vi "Oscilloscope_Analyzer.vi"(7 "Note":enum16{"Модулятор", "Команда", "Кадер", "Кодер"}(ring), 8 "error in (no error)":errorcluster, 11 "RFID system in":refnum<class "RFID system.lvclass">) -> (0 "error out":errorcluster, 3 "RFID system out":refnum<class "RFID system.lvclass">)   [LabVIEW 2019]
uses:
  <vilib>/express/express analysis/Spectral/XNode/ExpressSpectralMeasurementsBlockNode.xnode
  <vilib>/express/express analysis/Spectral/Block/exnSpectralBlock spectral measurements RMS poly.vi
  <vilib>/express/express analysis/Spectral/Block/exnSpectralBlock spectral measurements RMS WFM.vi
  Store.lvclass
  RFID system.lvclass
panel:
  in  "Tab Control":enum32{"Complex", "Real"}(tab)
  out "Osciloscope":cluster{"t0":dbl, "dt":dbl, "Y":dbl[]}(graph)
  out "Spectrum Analyzer":cluster{"t0":dbl, "dt":dbl, "Y":dbl[]}(graph)
  out "Osciloscope":waveform(dbl)(graph)
  out "Spectrum Analyzer":cluster{"t0":dbl, "dt":dbl, "Y":dbl[]}(graph)
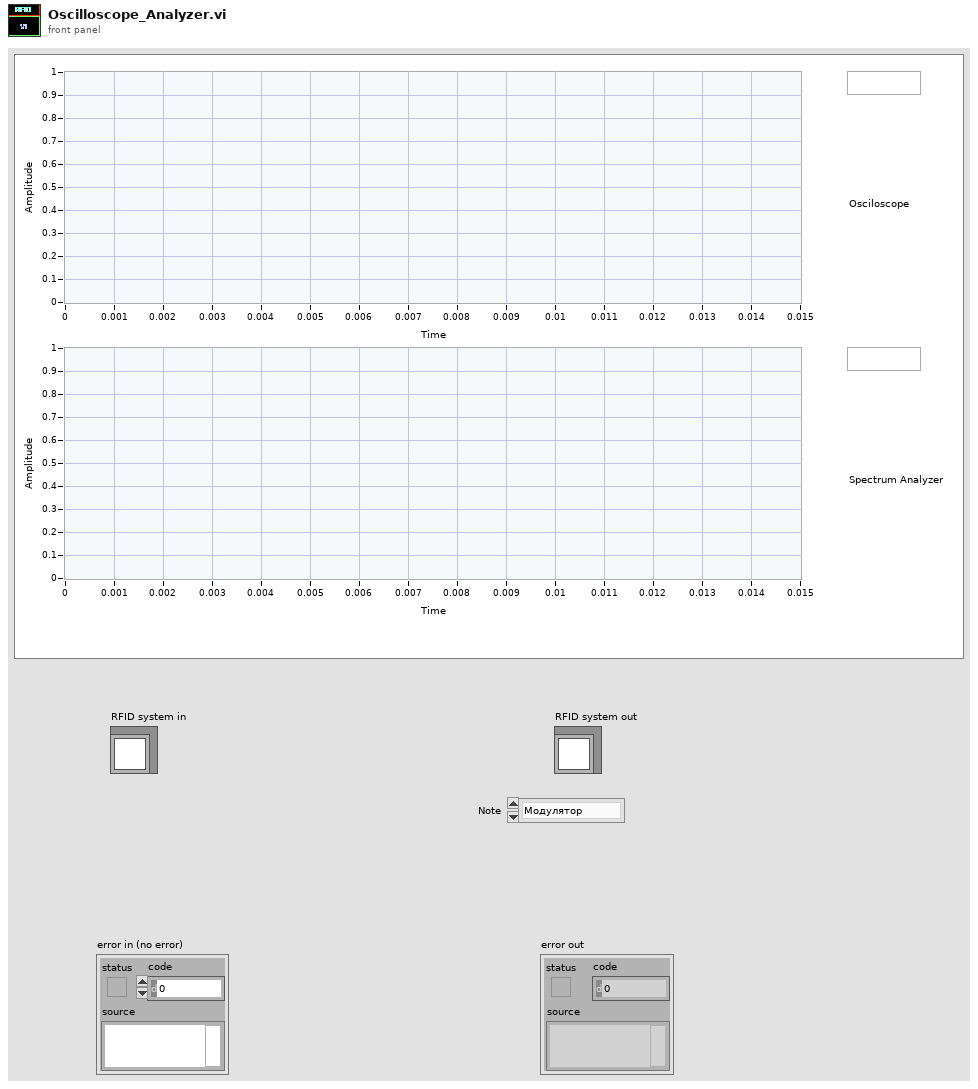
[diagram p1: front panel]
types:
  T1 = cluster{"averaging mode":u16, "weighting mode":u16, "number of averages":u32}
  T2 = cluster{"dB On (F)":bool, "unwrap phase (F)":bool, "convert to degree (F)":bool}
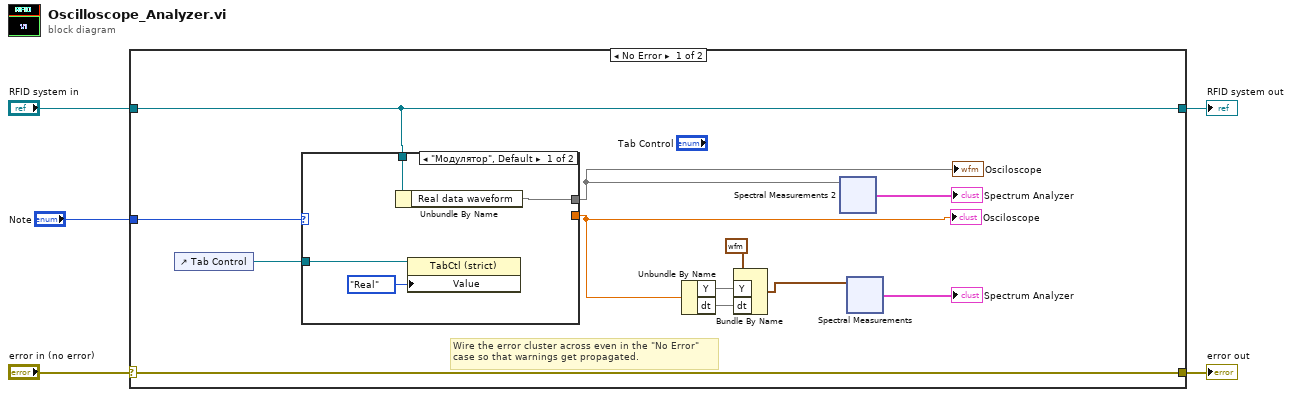
[diagram p0: block diagram]
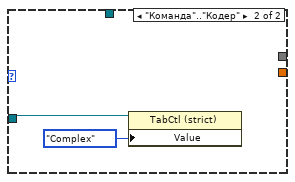
[diagram p2: hidden frame]
diagram:
  n1 = case shown="No Error" "error in (no error)" {
    selector: "error in (no error)" -> [w17 w47]
    tunnel: [w17 w47] -> w4
    tunnel: [w6 w46] -> w2
    tunnel: "RFID system in" -> [w6 w46]
    tunnel: "Note" -> [w16 _]
    frame No Error {
      # "Wire the error cluster across even in the \"No Error\"\ncase so that warnings get propagated."
      n2 = control-ref of="Tab Control"() -> (w9:refnum<vi>)
      n3 = case shown="\"Модулятор\", Default" w16 {
        tunnel: w6 -> [w41 w45]
        tunnel: [_ w44] -> w10
        tunnel: w9 -> [w40 w42]
        tunnel: [w38 _] -> w8
        frame "Модулятор", Default {
          n4 = Unbundle By Name(w41) -> ("Real data waveform"=w38)
          n5 = property class="TabCtl (strict)"(reference=w40, "Value"=enum32{"Complex", "Real"}."Real") -> ()  [unwired: 1 in, 2 out]
        }
        frame "Команда".."Кодер" {
          n6 = property class="TabCtl (strict)"(reference=w42, "Value"=enum32{"Complex", "Real"}."Complex") -> ()  [unwired: 1 in, 2 out]
        }
      }
      "Osciloscope" <- w10
      "Osciloscope" <- w8
      n7 = Unbundle By Name(w10) -> ("Y"=w13, "dt"=w12)
      n8 = Bundle By Name(cluster=waveform(cdb) {"t0"=timestamp(0 s since 1904-01-01), "dt"=1.0, "Y"=[]} ("waveform"), "Y"=w13, "dt"=w12) -> (w11:waveform(cdb))
      n9 = xnode ("Spectral Measurements 2")("Signals"=w8) -> ("FFT - (RMS)"=→"Spectrum Analyzer":cluster{"f0":dbl, "df":dbl, "magnitude":dbl[]})  [unwired: 1 in, 2 out]
      n10 = xnode ("Spectral Measurements")("Signals"=w11) -> ("FFT - (RMS)"=→"Spectrum Analyzer":cluster{"f0":dbl, "df":dbl, "magnitude":dbl[]})  [unwired: 1 in, 2 out]
    }
    frame Error {
    }
  }
  "error out" <- w4
  "RFID system out" <- w2
